vi "Read Recordset (DBVIEW).vi"(8 "error in":errorcluster, 9 "No. of rows":i32=-1, 11 "Recordset In":refnum<k7>) -> (0 "error out":errorcluster, 1 "graphical data":cluster{timestamp[], dbl[]}[](array[cluster]), 2 "tabular data":string[][](array[string]), 3 "Recordset Out":refnum<k7>, 4 "Rows Returned":i32)   [LabVIEW 2014, in "hse-db.lvlib" / "ADO-DB-Driver.lvlib"]
uses:
  ADO-DB-Driver.lvlib
panel:
  out "records read so far":i32
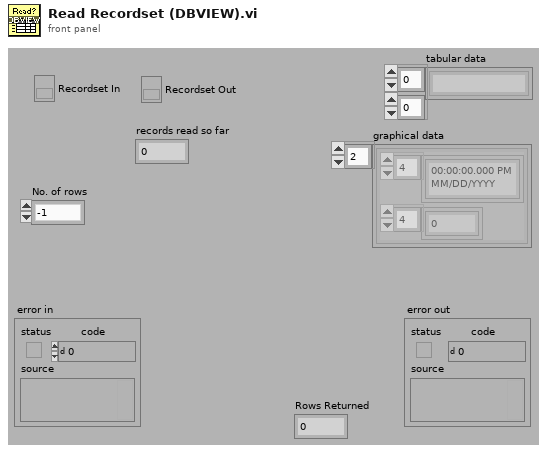
[diagram p1: front panel]
types:
  T1 = cluster{"timestamps":timestamp[], "values":dbl[]}[]
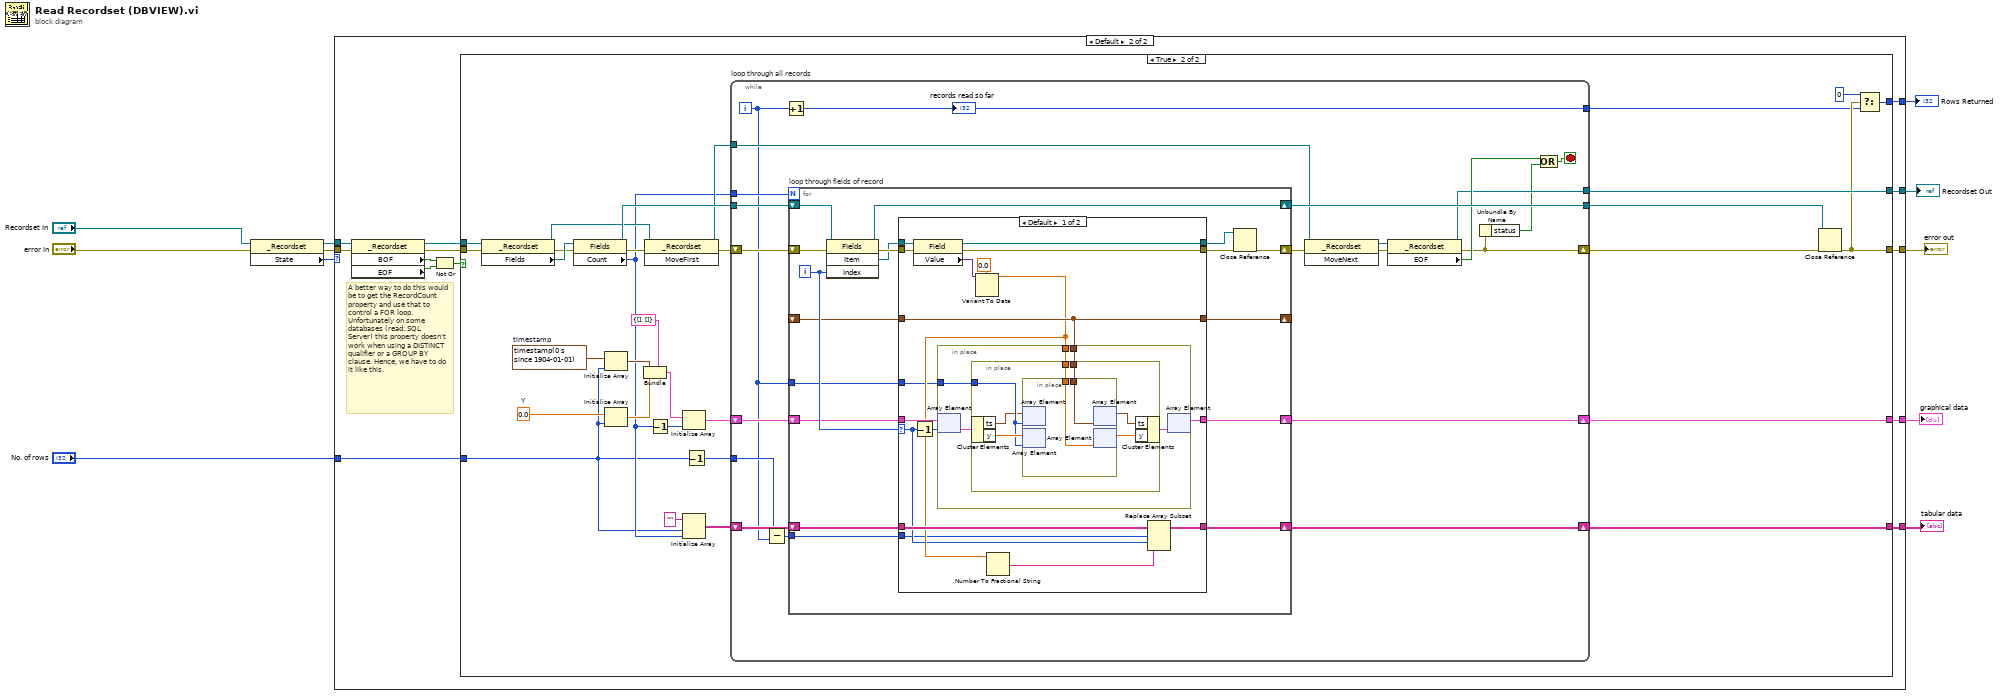
[diagram p0: block diagram]
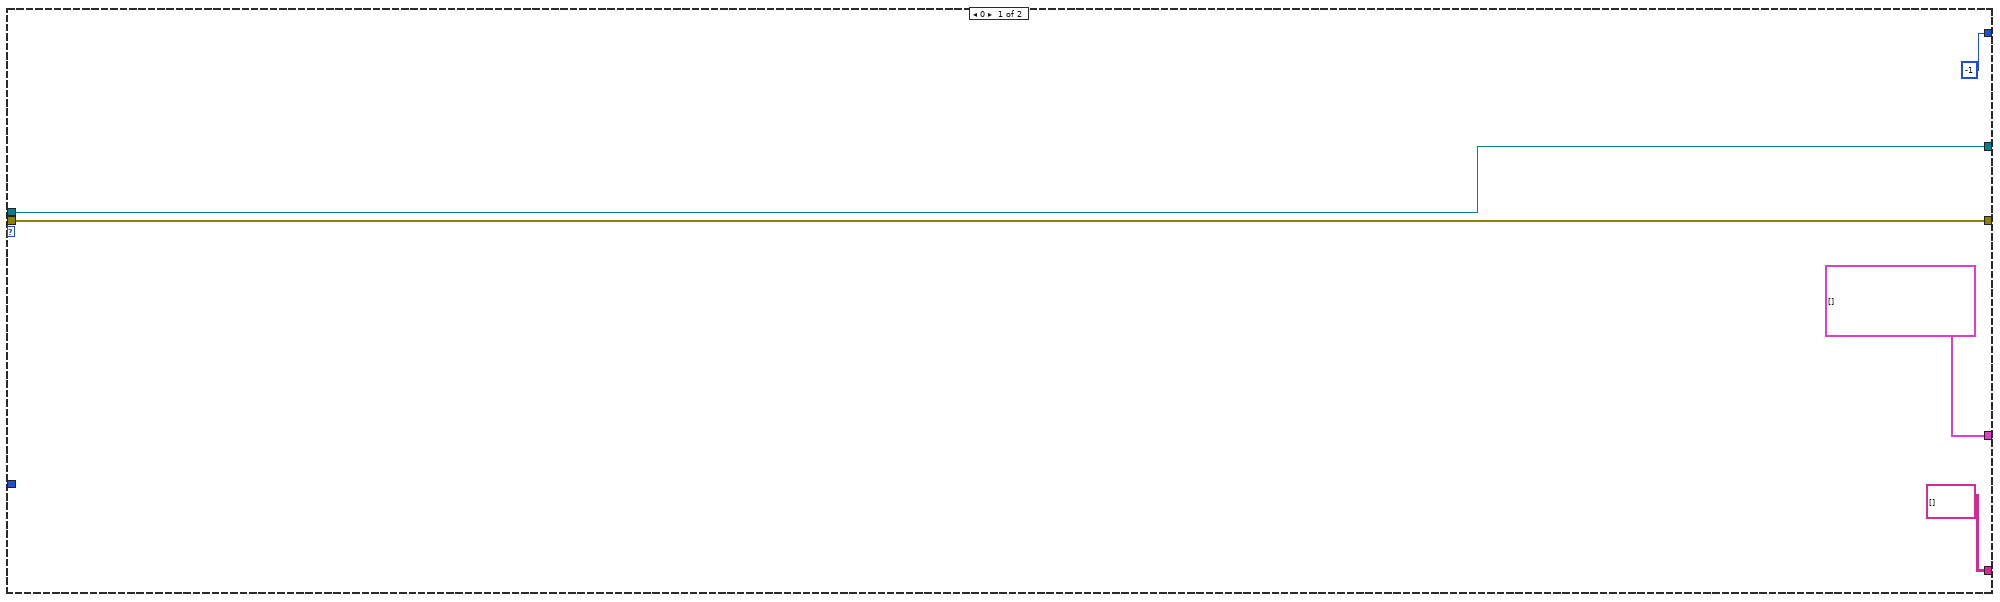
[diagram p2: hidden frame]
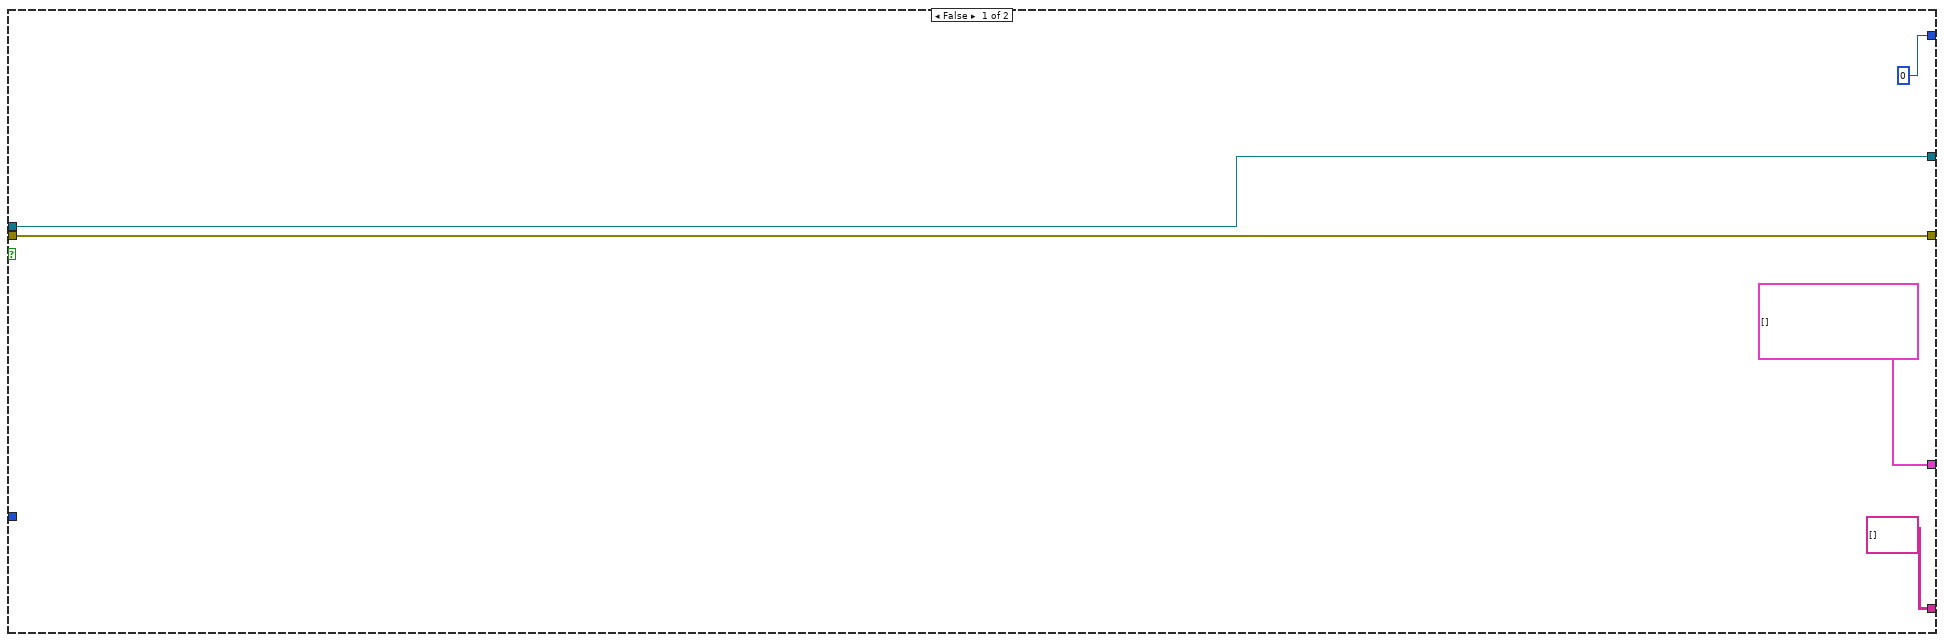
[diagram p3: hidden frame]
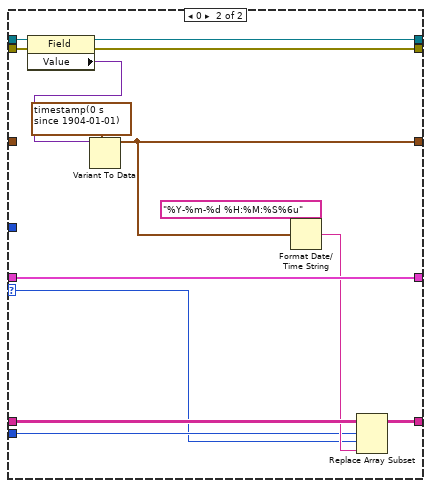
[diagram p4: hidden frame]
diagram:
  n1 = property class="_Recordset"(reference="Recordset In", error in="error in") -> (reference out=w8:refnum<k7>, error out=w6:errorcluster, "State"=w5:i32)
  n2 = case shown="Default" w5 {
    tunnel: [w14 w29] -> w11
    tunnel: [w16 w26] -> w4
    tunnel: [-1 w25] -> w10
    tunnel: w8 -> [w14 w21]
    tunnel: w6 -> [w16 w20]
    tunnel: [string[][] [] w19] -> w3
    tunnel: [T1 [] w18] -> w2
    tunnel: "No. of rows" -> [_ w17]
    frame 0 {
    }
    frame Default {
      # "A better way to do this would be to get the RecordCount property and use that to control a FOR loop. Unfortunately on some databases (read: SQL Server) this property doesn't work when using a DISTINCT qualifier or a GROUP BY clause. Hence, we have to do it like this."
      n3 = property class="_Recordset"(reference=w21, error in=w20) -> (reference out=w28:refnum<k7>, error out=w27:errorcluster, "BOF"=w24:bool, "EOF"=w22:bool)
      n4 = Not Or(1:w22, 2:w24) -> (0:w23:bool)
      n5 = case shown="True" w23 {
        tunnel: [w34 w65] -> w29
        tunnel: w28 -> [w34 w64]
        tunnel: w27 -> [w33 w63]
        tunnel: [w33 w61] -> w26
        tunnel: [0 ("Rows Returned") w62] -> w25
        tunnel: [string[][] [] w38] -> w19
        tunnel: [T1 [] w39] -> w18
        tunnel: w17 -> [_ w36]
        frame False {
        }
        frame True {
          w47 = 0.0  # Y
          w48 = timestamp(0 s since 1904-01-01)  # timestamp
          n6 = property class="_Recordset"(reference=w64, error in=w63) -> (reference out=w52:refnum<k7>, error out=w59:errorcluster, "Fields"=w60:refnum<k7>)
          n7 = property class="Fields"(reference=w60, error in=w59) -> (reference out=w57:refnum<k7>, error out=w55:errorcluster, "Count"=w37:i32)
          n8 = Initialize Array(w48, w36) -> (w46:timestamp[])
          n9 = Initialize Array(w47, w36) -> (w45:dbl[])
          n10 = Bundle(cluster=cluster{"ts":timestamp[], "y":dbl[]} {"ts"=[], "y"=[]}, "ts"=w46, "y"=w45) -> (w44:cluster{"ts":timestamp[], "y":dbl[]})
          n11 = invoke class="_Recordset" method="MoveFirst"(reference=w52, error in=w55) -> (reference out=w54:refnum<k7>, error out=w53:errorcluster)  [unwired: 1 in, 1 out]
          n12 = Decrement(x=w37) -> (x-1=w42:i32)
          n13 = Initialize Array(w44, w42) -> (w43:cluster{"ts":timestamp[], "y":dbl[]}[])
          n14 = Initialize Array("" ("Y"), w36, w37) -> (w49:string[][])
          n15 = Decrement(x=w36) -> (x-1=w35:i32)
          n16 = while "loop through all records" {
            shift-right: [w73] -> w58
            shift-left: w53 -> [w78]
            tunnel: w37 -> [w86]
            tunnel: [w81] -> w40
            tunnel: w54 -> [w79]
            tunnel: [w75] -> w65
            tunnel: w57 -> [w85]
            tunnel: [w84] -> w56
            shift-right: [w70] -> w39
            shift-left: w43 -> [w71]
            shift-right: [w69] -> w38
            shift-left: w49 -> [w72]
            tunnel: w35 -> [w68]
            i -> [w67]
            stop <- w83 stop-if-true
            n17 = Subtract(x=w68, y=w67) -> (x-y=w66:i32)
            n18 = Increment(x=w67) -> (x+1=w81:i32)
            "records read so far" <- w81
            n19 = for "loop through fields of record" {
              N: w86 -> [_]
              shift-right: [w97] -> w80
              shift-left: w78 -> [w102]
              shift-right: [w98] -> w84
              shift-left: w85 -> [w99]
              shift-right: [w93] -> w69
              shift-left: w72 -> [w94]
              shift-right: [w91] -> w70
              shift-left: w71 -> [w92]
              shift-right: [w90] -> _
              shift-left: _ -> [w89]
              tunnel: w67 -> [w88]
              tunnel: w66 -> [w87]
              i -> [w95]
              n20 = invoke class="Fields" method="Item"(reference=w99, error in=w102, "Index"=w95) -> (reference out=w98:refnum<k7>, error out=w103:errorcluster, "Item"=w96:refnum<k7>)  [unwired: 1 in, 1 out]
              n21 = case shown="Default" w95 {
                selector: w95 -> [w105 w135]
                tunnel: w103 -> [w120 w148]
                tunnel: [w119 w145] -> w101
                tunnel: [w118 w146] -> w100
                tunnel: w96 -> [w117 w147]
                tunnel: w94 -> [w115 w142]
                tunnel: [w114 w141] -> w93
                tunnel: w92 -> [w111 w138]
                tunnel: [w110 w138] -> w91
                tunnel: [w108 w139] -> w90
                tunnel: w89 -> [w108 _]
                tunnel: w88 -> [w106 _]
                tunnel: w87 -> [w104 w136]
                frame Default {
                  n22 = property class="Field"(reference=w117, error in=w120) -> (reference out=w119:refnum<k7>, error out=w118:errorcluster, "Value"=w112:variant)
                  n23 = Decrement(x=w105) -> (x-1=w109:i32)
                  n24 = Variant To Data(type=0.0 ("Y"), Variant=w112) -> (data=w107:dbl)  [unwired: 1 in, 1 out]
                  n25 = in-place {
                    in-place-border: w108 -> [w123]
                    in-place-border: w107 -> [w122]
                    in-place-border: w106 -> [w121]
                    n26 = in-place-array #1(w111, w109) -> (w125:cluster{"ts":timestamp[], "y":dbl[]})
                    n27 = in-place {
                      in-place-border: w123 -> [w129]
                      in-place-border: w122 -> [w128]
                      in-place-border: w121 -> [w127]
                      n28 = in-place-cluster #2(w125) -> ("ts"=w126:timestamp[], "y"=w132:dbl[])
                      n29 = in-place {
                        in-place-border: w129 -> [w134]
                        in-place-border: w128 -> [w133]
                        n30 = in-place-array #3(w126, w127) -> ()  [unwired: 1 out]
                        n31 = in-place-array #4(w132, w127) -> ()  [unwired: 1 out]
                        n32 = in-place-array #3(w134) -> (w131:timestamp[])  [unwired: 1 out]
                        n33 = in-place-array #4(w133) -> (w130:dbl[])  [unwired: 1 out]
                      }
                      n34 = in-place-cluster #2("ts"=w131, "y"=w130) -> (w124:cluster{"ts":timestamp[], "y":dbl[]})
                    }
                    n35 = in-place-array #1(w124) -> (w110:cluster{"ts":timestamp[], "y":dbl[]}[])  [unwired: 1 out]
                  }
                  n36 = Number To Fractional String(number=w107) -> (F-format string=w113:string)  [unwired: 3 in]
                  n37 = Replace Array Subset(array=w115, new element=w113, index (row)=w104, index (col)=w105) -> (w114:string[][])
                }
                frame 0 {
                  n38 = property class="Field"(reference=w147, error in=w148) -> (reference out=w145:refnum<k7>, error out=w146:errorcluster, "Value"=w140:variant)
                  n39 = Variant To Data(type=timestamp(0 s since 1904-01-01), Variant=w140) -> (data=w139:timestamp)  [unwired: 1 in, 1 out]
                  n40 = Format Date/Time String(time format string (%c)="%Y-%m-%d %H:%M:%S%6u", seconds (now)=w139) -> (date/time string=w137:string)  [unwired: 1 in]
                  n41 = Replace Array Subset(array=w142, new element=w137, index (row)=w136, index (col)=w135) -> (w141:string[][])
                }
              }
              n42 = Close Reference(reference=w101, error in (no error)=w100) -> (error out=w97:errorcluster)
            }
            n43 = invoke class="_Recordset" method="MoveNext"(reference=w79, error in=w80) -> (reference out=w77:refnum<k7>, error out=w76:errorcluster)  [unwired: 1 in, 1 out]
            n44 = property class="_Recordset"(reference=w77, error in=w76) -> (reference out=w75:refnum<k7>, error out=w73:errorcluster, "EOF"=w82:bool)
            n45 = Unbundle By Name(w73) -> ("status"=w74:bool)
            n46 = Compound Arithmetic op=OR(w82, w74) -> (w83:bool)
          }
          n47 = Close Reference(reference=w56, error in (no error)=w58) -> (error out=w61:errorcluster)
          n48 = Select(t=0, s=w61, f=w40) -> (s? t:f=w62:i32)
        }
      }
    }
  }
  "error out" <- w4
  "Rows Returned" <- w10
  "Recordset Out" <- w11
  "tabular data" <- w3
  "graphical data" <- w2
